vi "MonthToDate.vi"(9 "End Date":string="2014/9/24", 11 "From Date":string="2014/9/20") -> (1 "Table Control":string[][](table), 2 "output array":string[][](array[string]))   [LabVIEW 2012]
uses:
  <vilib>/addons/database/Auxilliary.llb/DB Tools Cursor Type.ctl
  Global1.vi
  <vilib>/addons/database/Connection.llb/DB Tools Open Connec (Path).vi
  <vilib>/addons/database/Connection.llb/Conn Execute.vi
  <vilib>/addons/database/Recordset.llb/Rec Fetch Recordset Data (R).vi
  <vilib>/addons/database/Recordset.llb/Rec Destroy - Connection.vi
  <vilib>/addons/database/_DB Variant To Data/Database Variant To Data.xnode
  <vilib>/addons/database/NI_Database_API.lvlib
panel:
  out "error out":errorcluster
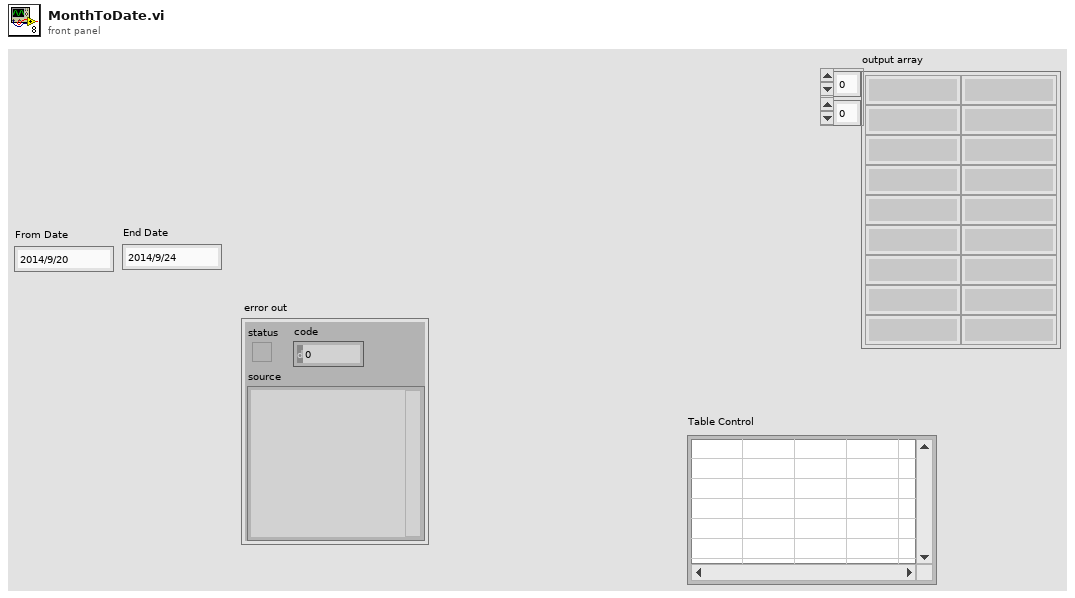
[diagram p1: front panel]
types:
  T1 = typedef "NI_Database_API.lvlib/DB Tools Cursor Type.ctl" = enum16{"forward-only", "keyset", "dynamic", "static"}
  T2 = typedef "NI_Database_API.lvlib/Conn ObjectReference.ctl" = refnum<k1>
  T3 = typedef "NI_Database_API.lvlib/Rec ObjectReference.ctl" = refnum<k1>
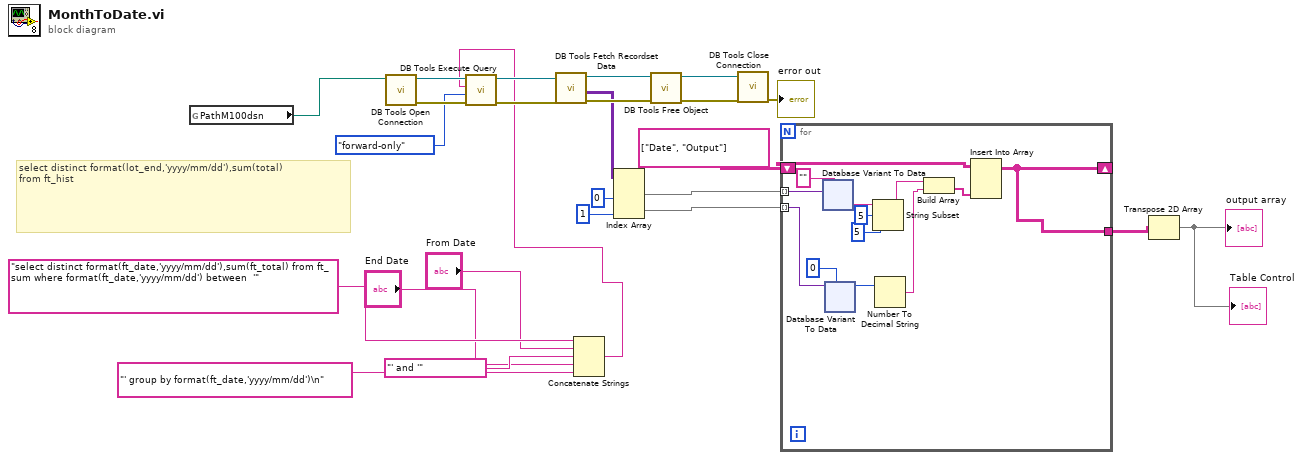
[diagram p0: block diagram]
diagram:
  # "select distinct format(lot_end,'yyyy/mm/dd'),sum(total)\nfrom ft_hist"
  n1 = global read "Global1.vi" "PathM100dsn"() -> (w1:path)
  n2 = call-poly <vilib>:"DB Tools Open Connection.vi"("connection information"=w1) -> ("error out"=w18:errorcluster, "connection reference"=w19:T2)  [unwired: 7 in]
  n3 = Concatenate Strings("select distinct format(ft_date,'yyyy/mm/dd'),sum(ft_total) from ft_sum where format(ft_date,'yyyy/mm/dd') between  '" ("SQL query"), "From Date", "' and '" ("string"), "End Date", "' group by format(ft_date,'yyyy/mm/dd')\n" ("string")) -> (w4:string)
  n4 = call-poly <vilib>:"DB Tools Execute Query.vi"("error in (no error)"=w18, "cursor type"=DB_Tools_Cursor_Type."forward-only", "SQL query"=w4, "connection reference"=w19) -> ("error out"=w20:errorcluster, "recordset reference"=w21:T3)  [unwired: 4 in]
  n5 = call-poly <vilib>:"DB Tools Fetch Recordset Data.vi"("error in (no error)"=w20, "recordset reference"=w21) -> ("error out"=w22:errorcluster, "recordset data"=w11:variant[][], "recordset reference out"=w23:T3)  [unwired: 3 in]
  n6 = Index Array(array=w11, index (col) #1=0 ("disabled index (col)"), index (col) #2=1 ("index (col)")) -> (element #1=w14:variant[], element #2=w13:variant[])  [unwired: 2 in]
  n7 = call-poly <vilib>:"DB Tools Free Object.vi"("error in (no error)"=w22, "recordset reference"=w23) -> ("error out"=w25:errorcluster, "connection reference"=w24:T2)  [unwired: 8 in]
  n8 = call <vilib>:"DB Tools Close Connection.vi"("error in (no error)"=w25, "connection reference"=w24) -> ("error out"=→"error out":errorcluster)  [unwired: 5 in]
  n9 = for {
    tunnel: w14 -> [w38] mode=indexing
    tunnel: w13 -> [w37] mode=indexing
    shift-right: [w31] -> _
    shift-left: string[][] [["Date", "Output"]] ("array") -> [w32]
    tunnel: [w31] -> w3
    n10 = xnode "Database Variant To Data"("database variant"=w38, "type"="") -> ("data"=w30:string)  [unwired: 1 in, 1 out]
    n11 = xnode "Database Variant To Data"("database variant"=w37, "type"=0) -> ("data"=w26:i32)  [unwired: 1 in, 1 out]
    n12 = String Subset(string=w30, offset (0)=5, length (rest)=5 ("length (rest)")) -> (substring=w29:string)
    n13 = Number To Decimal String(number=w26) -> (decimal integer string=w34:string)  [unwired: 1 in]
    n14 = Build Array(w29, w34) -> (w33:string[])
    n15 = Insert Into Array(array=w32, new element=w33) -> (w31:string[][])  [unwired: 2 in]
  }
  n16 = Transpose 2D Array(2D array=w3) -> (transposed array=→"output array" →"Table Control":string[][])
